vi "Engaging v2.vi"(6 "PID Cluster":T2={"L1 to L4 PID Cluster"={"L1 PID Gains"={"Kp"=0.005, "Kd"=0.5, "Ki"=0.0005}, "L2 PID Gains"={"Kp"=0.01, "Kd"=1.0, "Ki"=0.005}, "L3 PID Gains"={"Kp"=0.05, "Kd"=1.0, "Ki"=0.0005}, "L4 PID Gains"={"Kp"=0.1, "Kd"=0.1, "Ki"=0.0005}}, "Stage PID Cluster"={"Stage Z PID"={"Kp"=0.0005, "Kd"=0.001, "Ki"=0.0}, "Stage Y PID"={"Kp"=0.0003, "Kd"=0.01, "Ki"=0.0}, "Stage X PID"={"Kp"=0.0003, "Kd"=0.01, "Ki"=0.0}}, "OCT Z PID Gains"={"Kp"=0.0003, "Kd"=0.0001, "Ki"=0.01}}, 7 "Robot In":i32, 8 "error in":errorcluster, 9 "Engage Pt":dbl[](array[numeric])=[0.0, 0.0, 0.0, 0.0], 10 "Prev Posit Cluster":T3={"Prev L1 to L4 Posit"=[0.0, 0.0, 0.0, 0.0], "Prev Stage Posit"=[6.0, 6.0, 6.0], "Prev OCT Z Posit"=0.0}, 11 "FPGA VI Reference In":refnum<k20>) -> (0 "error out":errorcluster, 2 "Last Posit Cluster":T1={"Last L1 to L4 Posit"=[0.0, 0.0, 0.0, 0.0], "Last Stage Posit"=[6.0, 6.0, 6.0], "Last OCT Z Posit"=0.0}, 3 "FPGA VI Reference Out":refnum<k20>)   [LabVIEW 2016]
uses:
  Subsystems/Global Variables.vi
  <vilib>/Platform/TimedLoop/XDataNode/wakeup.ctl
  <vilib>/Platform/TimedLoop/XDataNode/XDNodeRunTimeDep.lvlib
  <vilib>/Platform/TimedLoop/XDataNode/nitl_modes.ctl
  <vilib>/Platform/TimedLoop/XDataNode/timing_clust.ctl
  <vilib>/platform/TimedLoop/XDataNode/XDataNode.xnode
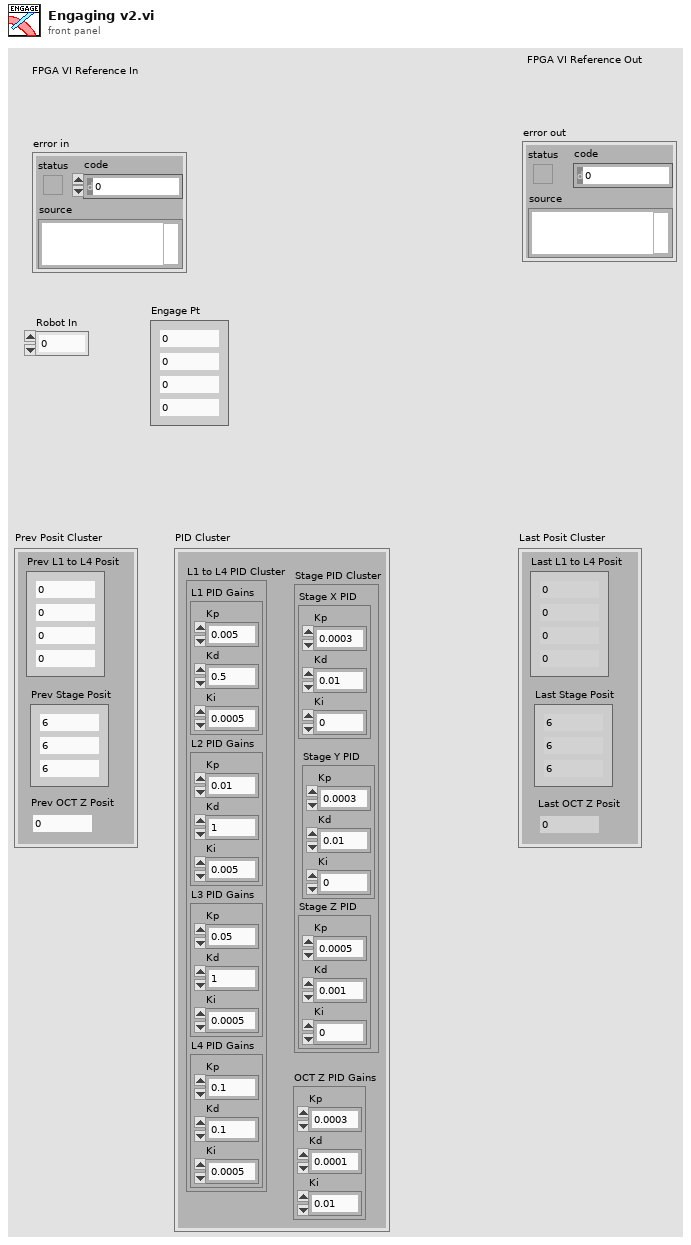
[diagram p1: front panel]
types:
  T1 = cluster{"Last L1 to L4 Posit":dbl[], "Last Stage Posit":dbl[], "Last OCT Z Posit":dbl}
  T2 = cluster{"L1 to L4 PID Cluster":cluster{"L1 PID Gains":cluster{"Kp":dbl, "Kd":dbl, "Ki":dbl}, "L2 PID Gains":cluster{"Kp":dbl, "Kd":dbl, "Ki":dbl}, "L3 PID Gains":cluster{"Kp":dbl, "Kd":dbl, "Ki":dbl}, "L4 PID Gains":cluster{"Kp":dbl, "Kd":dbl, "Ki":dbl}}, "Stage PID Cluster":cluster{"Stage Z PID":cluster{"Kp":dbl, "Kd":dbl, "Ki":dbl}, "Stage Y PID":cluster{"Kp":dbl, "Kd":dbl, "Ki":dbl}, "Stage X PID":cluster{"Kp":dbl, "Kd":dbl, "Ki":dbl}}, "OCT Z PID Gains":cluster{"Kp":dbl, "Kd":dbl, "Ki":dbl}}
  T3 = cluster{"Prev L1 to L4 Posit":dbl[], "Prev Stage Posit":dbl[], "Prev OCT Z Posit":dbl}
  T4 = typedef "XDNodeRunTimeDep.lvlib/timing_clust.ctl" = cluster{"Expected End [f-1]":u64, "Actual End [f-1]":u64, "Finished Late? [f-1]":bool, "Expected End [i-1]":u64, "Actual End [i-1]":u64, "Finished Late? [i-1]":bool, "Expected Start [i]":u64, "Actual Start [i]":u64, "Expected Start [f]":u64, "Actual Start [f]":u64, "Source Name":string, "Structure Name":string, "Period":i64, "Deadline":i64, "Offset":i64, "Start":i64, "Priority":i32, "Timeout":i32, "Mode":T5, "Wakeup Reason":T6, "Error":errorcluster, "Source Type":string, "Secondary Source Type":string, "Global End Time":u64, "Global Start Time":u64, "Frame Duration":u64, "Iteration Duration":u64, "Assigned CPU":i32, "I/O Scan Engine Mode":u32}
  T5 = typedef "XDNodeRunTimeDep.lvlib/nitl_modes.ctl" = enum32{"No Change", "Process missed periods, maintain original phase", "Discard missed periods, maintain original phase", "Process missed periods, ignore original phase", "Discard missed periods, ignore original phase"}
  T6 = typedef "XDNodeRunTimeDep.lvlib/wakeup.ctl" = enum32{"Normal", "Aborted", "Asynchronous wakeup", "Timing source error", "Timed loop error", "Timeout"}
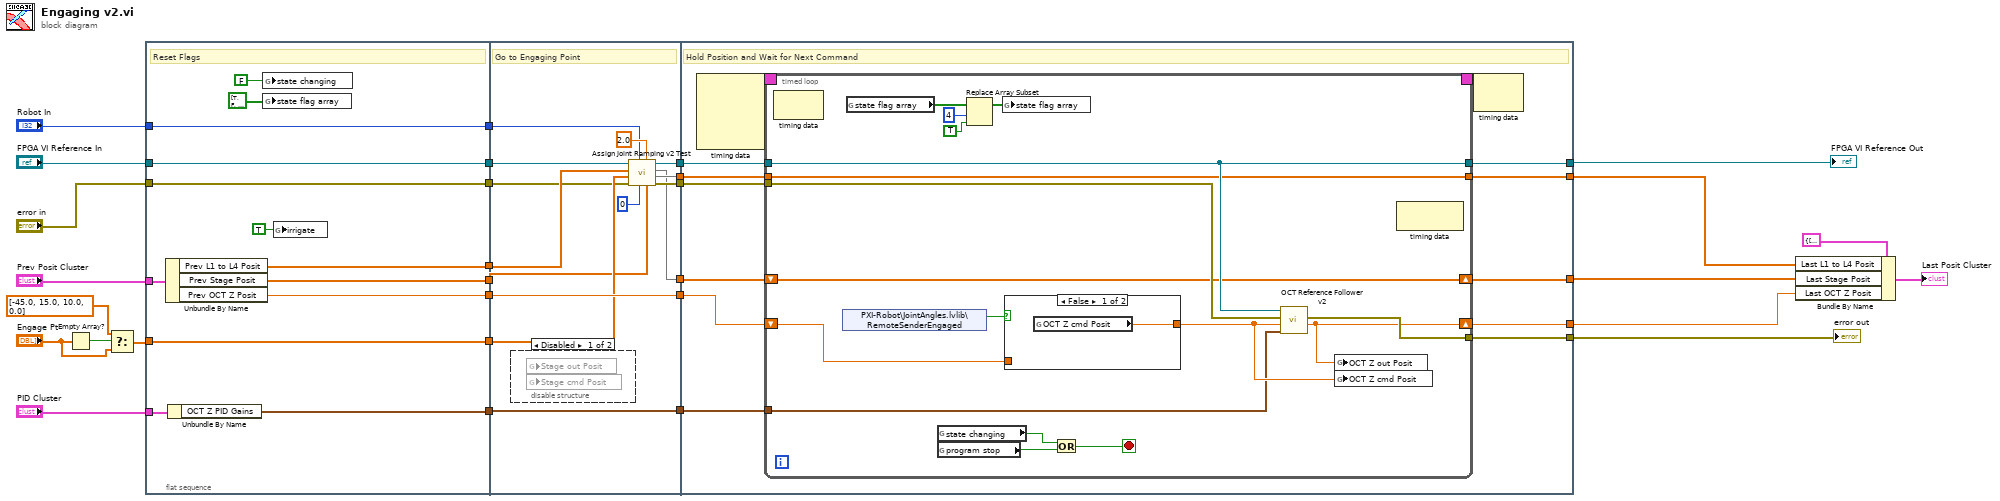
[diagram p0: block diagram]
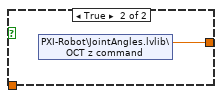
[diagram p3: hidden frame]
diagram:
  n1 = Empty Array?(array="Engage Pt") -> (empty?=w16:bool)
  n2 = Select(t=dbl[] [-45.0, 15.0, 10.0, 0.0] ("First Trk Pt 2"), s=w16, f="Engage Pt") -> (s? t:f=w13:dbl[])
  n3 = flat-sequence {
    tunnel: [w41] -> w30
    tunnel: "FPGA VI Reference In" -> [w41]
    tunnel: "error in" -> [w40]
    tunnel: [w40] -> w29
    tunnel: [w35] -> w28
    tunnel: "PID Cluster" -> [w34]
    tunnel: [w36] -> w27
    tunnel: w13 -> [w36]
    tunnel: "Prev Posit Cluster" -> [w39]
    tunnel: [w38] -> w26
    tunnel: [w37] -> w25
    tunnel: [w33] -> w24
    tunnel: "Robot In" -> [w32]
    tunnel: [w32] -> w1
    tunnel: w30 -> [w52]
    tunnel: w29 -> [w49]
    tunnel: w28 -> [w51]
    tunnel: w27 -> [w50]
    tunnel: [w53] -> w23
    tunnel: [w55] -> w22
    tunnel: [w56] -> w21
    tunnel: w26 -> [w45]
    tunnel: [w44] -> w20
    tunnel: [w57] -> w19
    tunnel: w25 -> [w57]
    tunnel: w24 -> [w56]
    tunnel: [w54] -> w18
    tunnel: w1 -> [w47]
    tunnel: [w66] -> w7
    tunnel: w23 -> [w67]
    tunnel: w22 -> [w68]
    tunnel: [w65] -> w11
    tunnel: [w64] -> w12
    tunnel: w21 -> [w63]
    tunnel: [w62] -> w8
    tunnel: [w61] -> w3
    tunnel: w20 -> [w60]
    tunnel: w19 -> [w59]
    tunnel: w18 -> [w58]
    frame #0 {
      # "Reset Flags"
      n4 = Unbundle By Name(w39) -> ("Prev L1 to L4 Posit"=w35:dbl[], "Prev Stage Posit"=w38:dbl[], "Prev OCT Z Posit"=w37:dbl)
      n5 = Unbundle By Name(w34) -> ("OCT Z PID Gains"=w33:cluster{"Kp":dbl, "Kd":dbl, "Ki":dbl})
      n6 = global write "Global Variables.vi" "state changing"(FALSE ("state changing")) -> ()
      n7 = global write "Global Variables.vi" "state flag array"(bool[] [TRUE, FALSE, FALSE, FALSE, FALSE, FALSE, FALSE, FALSE, FALSE] ("state flag array")) -> ()
      n8 = global write "Global Variables.vi" "irrigate"(TRUE ("irrigate")) -> ()
    }
    frame #1 {
      # "Go to Engaging Point"
      n9 = disable-structure shown="Disabled" {
        frame Disabled {
          n10 = global read "Global Variables.vi" "Stage out Posit"() -> ()  [unwired: 1 in]
          n11 = global read "Global Variables.vi" "Stage cmd Posit"() -> ()  [unwired: 1 in]
        }
        frame Enabled {
        }
      }
      n12 = call "Assign Joint Ramping v2 Test.vi"(4:w45, "Ramp Time [sec]"=2.0, "Vac Digital Cmd"=i8 0, "Robot In"=w47, "error in"=w49, "Destination Posit Array [mm]"=w50, 10:w51, "FPGA VI Reference In"=w52) -> ("error out"=w53:errorcluster, 1:w54, 2:w44, "FPGA VI Reference Out"=w55:refnum<k20>)
    }
    frame #2 {
      # "Hold Position and Wait for Next Command"
      n13 = node-c288() -> (w70:T4)  [unwired: 4 in]
      n14 = timed-loop {
        timing: w70 -> [_]
        timing-out: [_] -> w69
        tunnel: w68 -> [w75]
        tunnel: w67 -> [w74]
        tunnel: [w75] -> w66
        tunnel: [w73] -> w65
        tunnel: w63 -> [w78]
        tunnel: [w77] -> w61
        shift-right: [w71] -> w64
        shift-left: w60 -> [w71]
        shift-right: [w76] -> w62
        shift-left: w59 -> [w80]
        tunnel: w58 -> [w73]
        stop <- w81 stop-if-true
        n15 = node-c288() -> ()  [unwired: 1 in, 1 out]
        n16 = shared-variable "PXI-Robot\\JointAngles.lvlib\\RemoteSenderEngaged"() -> (w72:bool)  [unwired: 1 in, 1 out]
        n17 = global read "Global Variables.vi" "state flag array"() -> (w86:bool[])
        n18 = global read "Global Variables.vi" "state changing"() -> (w87:bool)
        n19 = global read "Global Variables.vi" "program stop"() -> (w82:bool)
        n20 = Replace Array Subset(array=w86, new element=TRUE ("new element/subarray"), index=4) -> (w85:bool[])
        n21 = global write "Global Variables.vi" "state flag array"(w85) -> ()
        n22 = case shown="False" w72 {
          tunnel: [w88 w89] -> w79
          tunnel: w80 -> [_ _]
          frame False {
            # "Hold Position if not Engaged"
            n23 = global read "Global Variables.vi" "OCT Z cmd Posit"() -> (w88:dbl)
          }
          frame True {
            n24 = shared-variable "PXI-Robot\\JointAngles.lvlib\\OCT z command"() -> (w89:dbl)  [unwired: 1 in, 1 out]
          }
        }
        n25 = Or(x=w87, y=w82) -> (x .or. y?=w81:bool)
        n26 = call "OCT Reference Follower v2.vi"("OCT Z PID Gains"=w78, "OCT  Z cmd Posit [mm]"=w79, "error in"=w74, "FPGA VI Reference In"=w75) -> ("OCT  Z out Posit [mm]"=w76:dbl, "error out"=w77:errorcluster)  [unwired: 5 in, 1 out]
        n27 = global write "Global Variables.vi" "OCT Z out Posit"(w76) -> ()
        n28 = global write "Global Variables.vi" "OCT Z cmd Posit"(w79) -> ()
        n29 = node-c288() -> ()  [unwired: 1 in, 1 out]
      }
      n30 = node-c288(w69) -> ()  [unwired: 1 out]
    }
  }
  n31 = Bundle By Name(cluster=T1 {"Last L1 to L4 Posit"=[0.0, 0.0, 0.0, 0.0], "Last Stage Posit"=[6.0, 6.0, 6.0], "Last OCT Z Posit"=0.0} ("Last Posit Cluster 2"), "Last L1 to L4 Posit"=w11, "Last Stage Posit"=w12, "Last OCT Z Posit"=w8) -> (→"Last Posit Cluster":T1)
  "FPGA VI Reference Out" <- w7
  "error out" <- w3
